vi "HEWH RLT Selected MW100 TCs.vi"(0 "Core HEWH Data Station A":T1={"Scan Rate Adjust"=0.0, "Draw Count"=0, "Test Patten Setup"={"Total Gallons Schedule"=[], "PRAT/RLT Sequence"=[{"Sequence #"=1.0, "Cycles"=35, "Mode Setting"="", "Flow Rate (GPM)"=0.0, "Temperature (F)"=0.0, "Reset Timer"=FALSE, "Use Temp Decline Method"=FALSE, "Terminate Condition"=enum."C1-Terminate Draw @ Gallon Mark", "Condition Value #1"=0.0, "UE"=FALSE, "LE"=FALSE, "Comp"=FALSE, "Fan"=FALSE, "Test End Time (Sec)"=0.0, "Purge Until Cutout"=FALSE, "Start Conditions"=enum."Heat Source Cutout", "Condition Value #2"=0.0, "Remove Power"=FALSE, "Time"=0.0, "Check Special Cond."=enum."SC2-Check Heat Source (On-C2/Off-C1)", "Condition#"=enum."C1", "Draw Flags"=enum."N/A", "Data Processing Delay (FHD 15sec, UEF 5 Sec)"=0.0, "Test Complete"=FALSE, "User Setpoint"=0.0, "Tank Setpoint"=0.0}, {"Sequence #"=2.0, "Cycles"=15, "Mode Setting"="", "Flow Rate (GPM)"=0.0, "Temperature (F)"=0.0, "Reset Timer"=FALSE, "Use Temp Decline Method"=FALSE, "Terminate Condition"=enum."C1-Terminate Draw @ Gallon Mark", "Condition Value #1"=0.0, "UE"=FALSE, "LE"=FALSE, "Comp"=FALSE, "Fan"=FALSE, "Test End Time (Sec)"=0.0, "Purge Until Cutout"=FALSE, "Start Conditions"=enum."Heat Source Cutout", "Condition Value #2"=0.0, "Remove Power"=FALSE, "Time"=0.0, "Check Special Cond."=enum."SC2-Check Heat Source (On-C2/Off-C1)", "Condition#"=enum."C1", "Draw Flags"=enum."N/A", "Data Processing Delay (FHD 15sec, UEF 5 Sec)"=0.0, "Test Complete"=FALSE, "User Setpoint"=0.0, "Tank Setpoint"=0.0}, {"Sequence #"=3.0, "Cycles"=35, "Mode Setting"="", "Flow Rate (GPM)"=0.0, "Temperature (F)"=0.0, "Reset Timer"=FALSE, "Use Temp Decline Method"=FALSE, "Terminate Condition"=enum."C1-Terminate Draw @ Gallon Mark", "Condition Value #1"=0.0, "UE"=FALSE, "LE"=FALSE, "Comp"=FALSE, "Fan"=FALSE, "Test End Time (Sec)"=0.0, "Purge Until Cutout"=FALSE, "Start Conditions"=enum."Heat Source Cutout", "Condition Value #2"=0.0, "Remove Power"=FALSE, "Time"=0.0, "Check Special Cond."=enum."SC2-Check Heat Source (On-C2/Off-C1)", "Condition#"=enum."C1", "Draw Flags"=enum."N/A", "Data Processing Delay (FHD 15sec, UEF 5 Sec)"=0.0, "Test Complete"=FALSE, "User Setpoint"=0.0, "Tank Setpoint"=0.0}, {"Sequence #"=4.0, "Cycles"=15, "Mode Setting"="", "Flow Rate (GPM)"=0.0, "Temperature (F)"=0.0, "Reset Timer"=FALSE, "Use Temp Decline Method"=FALSE, "Terminate Condition"=enum."C1-Terminate Draw @ Gallon Mark", "Condition Value #1"=0.0, "UE"=FALSE, "LE"=FALSE, "Comp"=FALSE, "Fan"=FALSE, "Test End Time (Sec)"=0.0, "Purge Until Cutout"=FALSE, "Start Conditions"=enum."Heat Source Cutout", "Condition Value #2"=0.0, "Remove Power"=FALSE, "Time"=0.0, "Check Special Cond."=enum."SC2-Check Heat Source (On-C2/Off-C1)", "Condition#"=enum."C1", "Draw Flags"=enum."N/A", "Data Processing Delay (FHD 15sec, UEF 5 Sec)"=0.0, "Test Complete"=FALSE, "User Setpoint"=0.0, "Tank Setpoint"=0.0}, {"Sequence #"=5.0, "Cycles"=35, "Mode Setting"="", "Flow Rate (GPM)"=0.0, "Temperature (F)"=0.0, "Reset Timer"=FALSE, "Use Temp Decline Method"=FALSE, "Terminate Condition"=enum."C1-Terminate Draw @ Gallon Mark", "Condition Value #1"=0.0, "UE"=FALSE, "LE"=FALSE, "Comp"=FALSE, "Fan"=FALSE, "Test End Time (Sec)"=0.0, "Purge Until Cutout"=FALSE, "Start Conditions"=enum."Heat Source Cutout", "Condition Value #2"=0.0, "Remove Power"=FALSE, "Time"=0.0, "Check Special Cond."=enum."SC2-Check Heat Source (On-C2/Off-C1)", "Condition#"=enum."C1", "Draw Flags"=enum."N/A", "Data Processing Delay (FHD 15sec, UEF 5 Sec)"=0.0, "Test Complete"=FALSE, "User Setpoint"=0.0, "Tank Setpoint"=0.0}, {"Sequence #"=6.0, "Cycles"=15, "Mode Setting"="", "Flow Rate (GPM)"=0.0, "Temperature (F)"=0.0, "Reset Timer"=FALSE, "Use Temp Decline Method"=FALSE, "Terminate Condition"=enum."C1-Terminate Draw @ Gallon Mark", "Condition Value #1"=0.0, "UE"=FALSE, "LE"=FALSE, "Comp"=FALSE, "Fan"=FALSE, "Test End Time (Sec)"=0.0, "Purge Until Cutout"=FALSE, "Start Conditions"=enum."Heat Source Cutout", "Condition Value #2"=0.0, "Remove Power"=FALSE, "Time"=0.0, "Check Special Cond."=enum."SC2-Check Heat Source (On-C2/Off-C1)", "Condition#"=enum."C1", "Draw Flags"=enum."N/A", "Data Processing Delay (FHD 15sec, UEF 5 Sec)"=0.0, "Test Complete"=FALSE, "User Setpoint"=0.0, "Tank Setpoint"=0.0}, {"Sequence #"=7.0, "Cycles"=35, "Mode Setting"="", "Flow Rate (GPM)"=0.0, "Temperature (F)"=0.0, "Reset Timer"=FALSE, "Use Temp Decline Method"=FALSE, "Terminate Condition"=enum."C1-Terminate Draw @ Gallon Mark", "Condition Value #1"=0.0, "UE"=FALSE, "LE"=FALSE, "Comp"=FALSE, "Fan"=FALSE, "Test End Time (Sec)"=0.0, "Purge Until Cutout"=FALSE, "Start Conditions"=enum."Heat Source Cutout", "Condition Value #2"=0.0, "Remove Power"=FALSE, "Time"=0.0, "Check Special Cond."=enum."SC2-Check Heat Source (On-C2/Off-C1)", "Condition#"=enum."C1", "Draw Flags"=enum."N/A", "Data Processing Delay (FHD 15sec, UEF 5 Sec)"=0.0, "Test Complete"=FALSE, "User Setpoint"=0.0, "Tank Setpoint"=0.0}, {"Sequence #"=8.0, "Cycles"=15, "Mode Setting"="", "Flow Rate (GPM)"=0.0, "Temperature (F)"=0.0, "Reset Timer"=FALSE, "Use Temp Decline Method"=FALSE, "Terminate Condition"=enum."C1-Terminate Draw @ Gallon Mark", "Condition Value #1"=0.0, "UE"=FALSE, "LE"=FALSE, "Comp"=FALSE, "Fan"=FALSE, "Test End Time (Sec)"=0.0, "Purge Until Cutout"=FALSE, "Start Conditions"=enum."Heat Source Cutout", "Condition Value #2"=0.0, "Remove Power"=FALSE, "Time"=0.0, "Check Special Cond."=enum."SC2-Check Heat Source (On-C2/Off-C1)", "Condition#"=enum."C1", "Draw Flags"=enum."N/A", "Data Processing Delay (FHD 15sec, UEF 5 Sec)"=0.0, "Test Complete"=FALSE, "User Setpoint"=0.0, "Tank Setpoint"=0.0}], "Current Sequence Index"=0}, "HEWH Specific DAQ"={"HEWH Data"={"HEWH Standard"={"Voltage (Volts)"=0.0, "Current (Amps)"=0.0, "Power (Watts)"=0.0, "WattHours (Wh)"=0.0, "TC Tree (AVG)"=0.0, "Flow Rate (GPM)"=0.0, "Gallons (Gal)"=0.0, "RTD Out (Deg F)"=0.0, "RTD In (Deg F)"=0.0, "RTD Amb (Deg F)"=0.0, "TC Down"=0.0, "UE Event Lead"=0, "LE Event Lead"=0, "TC 8"=0.0, "TC 9"=0.0, "TC 10"=0.0, "TC Tree Array (1-6)"=[], "TC 7"=0.0, "PSI 1"=0.0, "PSI 2"=0.0, "PSI 3"=0.0, "PSI 4"=0.0}, "PRAT"={"Power (Watts) A"=4192.0, "Power (Watts) B"=4192.0, "Power (Watts) C"=4192.0, "Power (Watts) D"=4192.0, "TC1"=0.0, "TC2"=0.0, "TC3"=0.0, "TC4"=0.0, "WattHours (Wh) A"=4192.0, "WattHours (Wh) B"=4192.0, "WattHours (Wh) C"=4192.0, "WattHours (Wh) D"=4192.0, "Ambient"=0.0, "Extra Temp"=0.0}, "Additional Power Data"={"Vthd"=236.2, "Frequency (Hz)"=236.2, "Apparent Power (VA)"=236.2, "Power Factor"=236.2, "Current Crest Factor"=236.2, "Voltage Crest Factor"=236.2, "Integration Time (sec)"=236.2}}, "Flow Valve % Open"=0.0, "Power State"={"UE"=FALSE, "LE"=FALSE, "COMP"=FALSE, "FANS"=FALSE}, "Power Analyzer"=enum."APLUS", "Flow Valve uA Output"=0, "Gallons Start (Gal)"=0.0, "PI Output"=0.0}, "Test Output Data"={"PreDraw Data Table"=[], "Data Table"=[], "MW100 TC Headers"=[]}, "Calc and Calibration"={"Mean SD Var Max Min Array"=[], "Draw Statistics (DBL)"=[], "Calibration Coefficients DBL"=[], "Start Gallons"=0.0, "Starting Temp Decline"=0.0, "K-Factor (Temperature)"=0.0, "All Draw Stats"=[], "RTD Terminate Value"=0.0, "K-Factor (Flow)"=0.0, "Intellifaucet Type"="", "Thermal Stabil Array"=[], "Gas Thermal Stabil Complete"=FALSE, "Therm Reset Cmpt 1"=FALSE, "Therm Reset Cmpt 2"=FALSE, "Last Flow Rate (Therm)"=0.0, "State"=enum."State 1", "Gas Thermal Time"=0.0, "Target Rate (Thermal)"=0.0, "Thermal - Final"=[], "State5 Gal Water"=0.0, "State 5 Gal Gas"=0.0, "Intellif Open < 1"=0.0, "Intellif Open < 1.7"=0.0, "Intellif Open < 2.2"=0.0, "Intellif Open > 2.2"=0.0, "End of Draw\nComparison"=[], "Temperature Decline Method"={"Previous Cycle Count"=0, "Previous Max Temp In"=0.0, "Previous Trigger In"=0, "Start Timer"=0.0, "first_iteration"=0.0}}, "Current Draw Time"=0.0, "LV Program"=enum."HEWH", "Station ID"=enum."A", "Current Cond"=enum."N/A", "Test Complete"=FALSE, "ANSI Rate"={"Array 1"=[], "Array 3"=[], "Array 2"=[], "Start ANSI"=FALSE, "ANSI Start Time"=0.0, "Restart ANSI"=FALSE, "15 Min ANSI Avg (BTU/hr)"=0.0, "20 Min ANSI Avg (BTU/hr)"=0.0, "25 Min ANSI Avg (BTU/hr)"=0.0, "Absolute Pressure"=0.0, "Gas Temperature"=0.0, "Volumetric Flow Rate"=0.0, "Mass Flow Rate"=0.0, "Array 4"=[], "Array 5"=[], "Gas Rate"=0.0, "15 Min Pres Avg (PSIA)"=0.0, "20 Min Pres Avg (PSIA)"=0.0, "25 Min Pres Avg (PSIA)"=0.0, "15 Min Temp Avg (°F) "=0.0, "20 Min Temp Avg (°F)"=0.0, "25 Min Temp Avg (°F)"=0.0, "15 Min Uncorrected Avg (CFH)"=0.0, "20 Min Uncorrected Avg (CFH)"=0.0, "25 Min Uncorrected Avg (CFH)"=0.0, "15 Min Corrected Avg (SCFH)"=0.0, "20 Min Corrected Avg (SCFH)"=0.0, "25 Min Corrected Avg (SCFH)"=0.0, "15 Min Complete"=FALSE, "20 Min Complete"=FALSE, "25 Min Complete"=FALSE, "Heating Value (BTU/ft³)"=0.0, "CO CO2 15 Min"=[], "CO CO2 20 Min"=[], "CO CO2 25 Min"=[], "CO CO2 Real Time"=[]}, "Module 4 Relay Status"={"INTELLIFAUCET TEMP(T)/FLOW(F) (CH 041)"=FALSE, "INTELLIFAUCET READY (CH 042)"=FALSE, "INTELLIFAUCET START (CH 043)"=FALSE, "INTELLIFAUCET STOP (CH 044)"=FALSE, "MAIN POWER RELAY (CH 047)"=FALSE, "NOT USED (CH 045)"=FALSE, "NOT USED (CH 046)"=FALSE, "PURGE VALVE RELAY (CH 048)"=FALSE, "OUTLET VALVE RELAY (CH 049)"=FALSE, "INLET VALVE RELAY (CH 050)"=FALSE, "Intellifaucet (% Open)"=0.0, "Proportioning Valve (%Open)"=0.0, "Intellifaucet Temp Setpoint (F)"=0.0}} {"Test Patten Setup"."PRAT/RLT Sequence"."Time" format="%<%H:%M:%S>t"; "Test Patten Setup"."Total Gallons Schedule" format="%.2f"}, 1 "Current Drawing Station":string="A", 2 "Show Flow Data":bool, 9 "MW100 Full Data":string[][](array[string])=[["Voltage (V)", "0.000"], ["RMS Current (Amps)", "0.000"], ["Power (Watts)", "0.000"], ["Watt Hours (Wh)", "0.000"], ["Voltage Total Harmonic Distortion", "0.000"], ["Frequency (Hz)", "0.000"], ["Apparent Power (VA)", "0.000"], ["Power Factor", "0.000"], ["Current Crest Factor", "0.000"], ["Voltage Crest Factor", "0.000"], ["Integration Time (sec)", "0.000"], ["Intellifaucet Valve % Open", "0.000"], ["Draw Count", "1"], ["T1", "10.2"], ["T2", "20"], ["T3", "0.000"], ["T4", "0.000"], ["T5", "0.000"], ["T6", "0.000"], ["T7", "0.000"], ["T8", "0.000"], ["T9", "0.000"], ["T10", "0.000"], ["TC Tree Average", "0.000"], ["TC Down", "0.000"], ["RTD IN", "0.000"], ["RTD Out", "0.000"], ["RTD Ambient", "0.000"], ["Totalized Flow (Linear Link) - Calculated (Gallons)", "0.000"], ["Flow Rate (Linear Link) - Calculated (GPM)", "0.000"], ["Pressure - HI1", "0.000"], ["Pressure - HI2", "0.000"], ["Pressure - LOW", "0.000"], ["Pressure - PIN", "0.000"]], 11 "Error In":errorcluster, 12 "Station A Channels, MW100":string[][](array[string])=[["T1 - IN", "11"], ["T1 - OUT", "13"]], 13 "Station ID":string="A", 14 "Collect Power Data":bool) -> (3 "Data (Label,Data)":string[][](array[string])=[["Voltage (V)", "0.000"], ["RMS Current (Amps)", "0.000"], ["Power (Watts)", "0.000"], ["Watt Hours (Wh)", "0.000"], ["Voltage Total Harmonic Distortion", "0.000"], ["Frequency (Hz)", "0.000"], ["Apparent Power (VA)", "0.000"], ["Power Factor", "0.000"], ["Current Crest Factor", "0.000"], ["Voltage Crest Factor", "0.000"], ["Integration Time (sec)", "0.000"], ["Intellifaucet Valve % Open", "0.000"], ["TC Tree Average", "0.000"], ["TC Down", "0.000"], ["RTD IN", "0.000"], ["RTD Out", "0.000"], ["RTD Ambient", "0.000"], ["Totalized Flow (Linear Link) - Calculated (Gallons)", "0.000"], ["Flow Rate (Linear Link) - Calculated (GPM)", "0.000"], ["Pressure - HI1", "0.000"], ["Pressure - HI2", "0.000"], ["Pressure - LOW", "0.000"], ["Pressure - PIN", "0.000"]], 4 "Core HEWH Data Station Output":T1={"Scan Rate Adjust"=0.0, "Draw Count"=0, "Test Patten Setup"={"Total Gallons Schedule"=[], "PRAT/RLT Sequence"=[{"Sequence #"=1.0, "Cycles"=35, "Mode Setting"="", "Flow Rate (GPM)"=0.0, "Temperature (F)"=0.0, "Reset Timer"=FALSE, "Use Temp Decline Method"=FALSE, "Terminate Condition"=enum."C1-Terminate Draw @ Gallon Mark", "Condition Value #1"=0.0, "UE"=FALSE, "LE"=FALSE, "Comp"=FALSE, "Fan"=FALSE, "Test End Time (Sec)"=0.0, "Purge Until Cutout"=FALSE, "Start Conditions"=enum."Heat Source Cutout", "Condition Value #2"=0.0, "Remove Power"=FALSE, "Time"=0.0, "Check Special Cond."=enum."SC2-Check Heat Source (On-C2/Off-C1)", "Condition#"=enum."C1", "Draw Flags"=enum."N/A", "Data Processing Delay (FHD 15sec, UEF 5 Sec)"=0.0, "Test Complete"=FALSE, "User Setpoint"=0.0, "Tank Setpoint"=0.0}, {"Sequence #"=2.0, "Cycles"=15, "Mode Setting"="", "Flow Rate (GPM)"=0.0, "Temperature (F)"=0.0, "Reset Timer"=FALSE, "Use Temp Decline Method"=FALSE, "Terminate Condition"=enum."C1-Terminate Draw @ Gallon Mark", "Condition Value #1"=0.0, "UE"=FALSE, "LE"=FALSE, "Comp"=FALSE, "Fan"=FALSE, "Test End Time (Sec)"=0.0, "Purge Until Cutout"=FALSE, "Start Conditions"=enum."Heat Source Cutout", "Condition Value #2"=0.0, "Remove Power"=FALSE, "Time"=0.0, "Check Special Cond."=enum."SC2-Check Heat Source (On-C2/Off-C1)", "Condition#"=enum."C1", "Draw Flags"=enum."N/A", "Data Processing Delay (FHD 15sec, UEF 5 Sec)"=0.0, "Test Complete"=FALSE, "User Setpoint"=0.0, "Tank Setpoint"=0.0}, {"Sequence #"=3.0, "Cycles"=35, "Mode Setting"="", "Flow Rate (GPM)"=0.0, "Temperature (F)"=0.0, "Reset Timer"=FALSE, "Use Temp Decline Method"=FALSE, "Terminate Condition"=enum."C1-Terminate Draw @ Gallon Mark", "Condition Value #1"=0.0, "UE"=FALSE, "LE"=FALSE, "Comp"=FALSE, "Fan"=FALSE, "Test End Time (Sec)"=0.0, "Purge Until Cutout"=FALSE, "Start Conditions"=enum."Heat Source Cutout", "Condition Value #2"=0.0, "Remove Power"=FALSE, "Time"=0.0, "Check Special Cond."=enum."SC2-Check Heat Source (On-C2/Off-C1)", "Condition#"=enum."C1", "Draw Flags"=enum."N/A", "Data Processing Delay (FHD 15sec, UEF 5 Sec)"=0.0, "Test Complete"=FALSE, "User Setpoint"=0.0, "Tank Setpoint"=0.0}, {"Sequence #"=4.0, "Cycles"=15, "Mode Setting"="", "Flow Rate (GPM)"=0.0, "Temperature (F)"=0.0, "Reset Timer"=FALSE, "Use Temp Decline Method"=FALSE, "Terminate Condition"=enum."C1-Terminate Draw @ Gallon Mark", "Condition Value #1"=0.0, "UE"=FALSE, "LE"=FALSE, "Comp"=FALSE, "Fan"=FALSE, "Test End Time (Sec)"=0.0, "Purge Until Cutout"=FALSE, "Start Conditions"=enum."Heat Source Cutout", "Condition Value #2"=0.0, "Remove Power"=FALSE, "Time"=0.0, "Check Special Cond."=enum."SC2-Check Heat Source (On-C2/Off-C1)", "Condition#"=enum."C1", "Draw Flags"=enum."N/A", "Data Processing Delay (FHD 15sec, UEF 5 Sec)"=0.0, "Test Complete"=FALSE, "User Setpoint"=0.0, "Tank Setpoint"=0.0}, {"Sequence #"=5.0, "Cycles"=35, "Mode Setting"="", "Flow Rate (GPM)"=0.0, "Temperature (F)"=0.0, "Reset Timer"=FALSE, "Use Temp Decline Method"=FALSE, "Terminate Condition"=enum."C1-Terminate Draw @ Gallon Mark", "Condition Value #1"=0.0, "UE"=FALSE, "LE"=FALSE, "Comp"=FALSE, "Fan"=FALSE, "Test End Time (Sec)"=0.0, "Purge Until Cutout"=FALSE, "Start Conditions"=enum."Heat Source Cutout", "Condition Value #2"=0.0, "Remove Power"=FALSE, "Time"=0.0, "Check Special Cond."=enum."SC2-Check Heat Source (On-C2/Off-C1)", "Condition#"=enum."C1", "Draw Flags"=enum."N/A", "Data Processing Delay (FHD 15sec, UEF 5 Sec)"=0.0, "Test Complete"=FALSE, "User Setpoint"=0.0, "Tank Setpoint"=0.0}, {"Sequence #"=6.0, "Cycles"=15, "Mode Setting"="", "Flow Rate (GPM)"=0.0, "Temperature (F)"=0.0, "Reset Timer"=FALSE, "Use Temp Decline Method"=FALSE, "Terminate Condition"=enum."C1-Terminate Draw @ Gallon Mark", "Condition Value #1"=0.0, "UE"=FALSE, "LE"=FALSE, "Comp"=FALSE, "Fan"=FALSE, "Test End Time (Sec)"=0.0, "Purge Until Cutout"=FALSE, "Start Conditions"=enum."Heat Source Cutout", "Condition Value #2"=0.0, "Remove Power"=FALSE, "Time"=0.0, "Check Special Cond."=enum."SC2-Check Heat Source (On-C2/Off-C1)", "Condition#"=enum."C1", "Draw Flags"=enum."N/A", "Data Processing Delay (FHD 15sec, UEF 5 Sec)"=0.0, "Test Complete"=FALSE, "User Setpoint"=0.0, "Tank Setpoint"=0.0}, {"Sequence #"=7.0, "Cycles"=35, "Mode Setting"="", "Flow Rate (GPM)"=0.0, "Temperature (F)"=0.0, "Reset Timer"=FALSE, "Use Temp Decline Method"=FALSE, "Terminate Condition"=enum."C1-Terminate Draw @ Gallon Mark", "Condition Value #1"=0.0, "UE"=FALSE, "LE"=FALSE, "Comp"=FALSE, "Fan"=FALSE, "Test End Time (Sec)"=0.0, "Purge Until Cutout"=FALSE, "Start Conditions"=enum."Heat Source Cutout", "Condition Value #2"=0.0, "Remove Power"=FALSE, "Time"=0.0, "Check Special Cond."=enum."SC2-Check Heat Source (On-C2/Off-C1)", "Condition#"=enum."C1", "Draw Flags"=enum."N/A", "Data Processing Delay (FHD 15sec, UEF 5 Sec)"=0.0, "Test Complete"=FALSE, "User Setpoint"=0.0, "Tank Setpoint"=0.0}, {"Sequence #"=8.0, "Cycles"=15, "Mode Setting"="", "Flow Rate (GPM)"=0.0, "Temperature (F)"=0.0, "Reset Timer"=FALSE, "Use Temp Decline Method"=FALSE, "Terminate Condition"=enum."C1-Terminate Draw @ Gallon Mark", "Condition Value #1"=0.0, "UE"=FALSE, "LE"=FALSE, "Comp"=FALSE, "Fan"=FALSE, "Test End Time (Sec)"=0.0, "Purge Until Cutout"=FALSE, "Start Conditions"=enum."Heat Source Cutout", "Condition Value #2"=0.0, "Remove Power"=FALSE, "Time"=0.0, "Check Special Cond."=enum."SC2-Check Heat Source (On-C2/Off-C1)", "Condition#"=enum."C1", "Draw Flags"=enum."N/A", "Data Processing Delay (FHD 15sec, UEF 5 Sec)"=0.0, "Test Complete"=FALSE, "User Setpoint"=0.0, "Tank Setpoint"=0.0}], "Current Sequence Index"=0}, "HEWH Specific DAQ"={"HEWH Data"={"HEWH Standard"={"Voltage (Volts)"=0.0, "Current (Amps)"=0.0, "Power (Watts)"=0.0, "WattHours (Wh)"=0.0, "TC Tree (AVG)"=0.0, "Flow Rate (GPM)"=0.0, "Gallons (Gal)"=0.0, "RTD Out (Deg F)"=0.0, "RTD In (Deg F)"=0.0, "RTD Amb (Deg F)"=0.0, "TC Down"=0.0, "UE Event Lead"=0, "LE Event Lead"=0, "TC 8"=0.0, "TC 9"=0.0, "TC 10"=0.0, "TC Tree Array (1-6)"=[], "TC 7"=0.0, "PSI 1"=0.0, "PSI 2"=0.0, "PSI 3"=0.0, "PSI 4"=0.0}, "PRAT"={"Power (Watts) A"=4192.0, "Power (Watts) B"=4192.0, "Power (Watts) C"=4192.0, "Power (Watts) D"=4192.0, "TC1"=0.0, "TC2"=0.0, "TC3"=0.0, "TC4"=0.0, "WattHours (Wh) A"=4192.0, "WattHours (Wh) B"=4192.0, "WattHours (Wh) C"=4192.0, "WattHours (Wh) D"=4192.0, "Ambient"=0.0, "Extra Temp"=0.0}, "Additional Power Data"={"Vthd"=236.2, "Frequency (Hz)"=236.2, "Apparent Power (VA)"=236.2, "Power Factor"=236.2, "Current Crest Factor"=236.2, "Voltage Crest Factor"=236.2, "Integration Time (sec)"=236.2}}, "Flow Valve % Open"=0.0, "Power State"={"UE"=FALSE, "LE"=FALSE, "COMP"=FALSE, "FANS"=FALSE}, "Power Analyzer"=enum."APLUS", "Flow Valve uA Output"=0, "Gallons Start (Gal)"=0.0, "PI Output"=0.0}, "Test Output Data"={"PreDraw Data Table"=[], "Data Table"=[], "MW100 TC Headers"=[]}, "Calc and Calibration"={"Mean SD Var Max Min Array"=[], "Draw Statistics (DBL)"=[], "Calibration Coefficients DBL"=[], "Start Gallons"=0.0, "Starting Temp Decline"=0.0, "K-Factor (Temperature)"=0.0, "All Draw Stats"=[], "RTD Terminate Value"=0.0, "K-Factor (Flow)"=0.0, "Intellifaucet Type"="", "Thermal Stabil Array"=[], "Gas Thermal Stabil Complete"=FALSE, "Therm Reset Cmpt 1"=FALSE, "Therm Reset Cmpt 2"=FALSE, "Last Flow Rate (Therm)"=0.0, "State"=enum."State 1", "Gas Thermal Time"=0.0, "Target Rate (Thermal)"=0.0, "Thermal - Final"=[], "State5 Gal Water"=0.0, "State 5 Gal Gas"=0.0, "Intellif Open < 1"=0.0, "Intellif Open < 1.7"=0.0, "Intellif Open < 2.2"=0.0, "Intellif Open > 2.2"=0.0, "End of Draw\nComparison"=[], "Temperature Decline Method"={"Previous Cycle Count"=0, "Previous Max Temp In"=0.0, "Previous Trigger In"=0, "Start Timer"=0.0, "first_iteration"=0.0}}, "Current Draw Time"=0.0, "LV Program"=enum."HEWH", "Station ID"=enum."A", "Current Cond"=enum."N/A", "Test Complete"=FALSE, "ANSI Rate"={"Array 1"=[], "Array 3"=[], "Array 2"=[], "Start ANSI"=FALSE, "ANSI Start Time"=0.0, "Restart ANSI"=FALSE, "15 Min ANSI Avg (BTU/hr)"=0.0, "20 Min ANSI Avg (BTU/hr)"=0.0, "25 Min ANSI Avg (BTU/hr)"=0.0, "Absolute Pressure"=0.0, "Gas Temperature"=0.0, "Volumetric Flow Rate"=0.0, "Mass Flow Rate"=0.0, "Array 4"=[], "Array 5"=[], "Gas Rate"=0.0, "15 Min Pres Avg (PSIA)"=0.0, "20 Min Pres Avg (PSIA)"=0.0, "25 Min Pres Avg (PSIA)"=0.0, "15 Min Temp Avg (°F) "=0.0, "20 Min Temp Avg (°F)"=0.0, "25 Min Temp Avg (°F)"=0.0, "15 Min Uncorrected Avg (CFH)"=0.0, "20 Min Uncorrected Avg (CFH)"=0.0, "25 Min Uncorrected Avg (CFH)"=0.0, "15 Min Corrected Avg (SCFH)"=0.0, "20 Min Corrected Avg (SCFH)"=0.0, "25 Min Corrected Avg (SCFH)"=0.0, "15 Min Complete"=FALSE, "20 Min Complete"=FALSE, "25 Min Complete"=FALSE, "Heating Value (BTU/ft³)"=0.0, "CO CO2 15 Min"=[], "CO CO2 20 Min"=[], "CO CO2 25 Min"=[], "CO CO2 Real Time"=[]}, "Module 4 Relay Status"={"INTELLIFAUCET TEMP(T)/FLOW(F) (CH 041)"=FALSE, "INTELLIFAUCET READY (CH 042)"=FALSE, "INTELLIFAUCET START (CH 043)"=FALSE, "INTELLIFAUCET STOP (CH 044)"=FALSE, "MAIN POWER RELAY (CH 047)"=FALSE, "NOT USED (CH 045)"=FALSE, "NOT USED (CH 046)"=FALSE, "PURGE VALVE RELAY (CH 048)"=FALSE, "OUTLET VALVE RELAY (CH 049)"=FALSE, "INLET VALVE RELAY (CH 050)"=FALSE, "Intellifaucet (% Open)"=0.0, "Proportioning Valve (%Open)"=0.0, "Intellifaucet Temp Setpoint (F)"=0.0}} {"Test Patten Setup"."PRAT/RLT Sequence"."Time" format="%<%H:%M:%S>t"; "Test Patten Setup"."Total Gallons Schedule" format="%.2f"}, 8 "RMS Current (Amps)":dbl, 10 "TC Data":string[][](array[string]), 15 "Error Out":errorcluster)   [LabVIEW 2023]
uses:
  Type Definitions/HEWH Output Information.ctl
  Type Definitions/HEWH Draw Pattern Setup.ctl
  Type Definitions/PRAT Test.ctl
  Utility/Save File/File Setup (Public)/Type Definition/Save File HEWH Heating Control Mode.ctl
  Draw Water Specific/Type Definitions/Terminate Draw Conditions.ctl
  Type Definitions/HEWH Start Conditions.ctl
  Draw Water Specific/Type Definitions/Check Special Condtions.ctl
  Draw Water Specific/Type Definitions/HEWH Special Condition Check.ctl
  Type Definitions/HEWH Draw Flag ENUM.ctl
  Type Definitions/HEWH Specific DAQ.ctl
  Type Definitions/HEWH Power Data.ctl
  Type Definitions/HEWH Power Elements.ctl
  Utility/Type Definitions/UTILITY Power Analyzer.ctl
  Type Definitions/HEWH Calc and Calibration.ctl
  Utility/Save File/File Setup (Public)/Type Definition/Save File DOE LabView Program.ctl
  Custom Instrument Control/MW100/Type Definitions/Station ID Selector.ctl
  Range/Type Definitions/RANGE ANSI Rate.ctl
  Custom Instrument Control/MW100/Type Definitions/HEWH Module 4 Relay Status.ctl
  Type Definitions/PRAT Channel Settings.ctl
  Custom Instrument Control/MW100/Type Definitions/HEWH MW100 Channel Numbers.ctl
  Utility/Save File/File Setup.lvlib
panel:
  out "All Other Data (NO TC's)":string[][](array[string])
  in  "PRAT Example Data":string[][](array[string])=[["Power (Watts) - Station A", "1"], ["Power (Watts) - Station B", "2"], ["Power (Watts) - Station C", "3"], ["Power (Watts) - Station D", "4"], ["WattHours (Wh) - Station A", "1"], ["WattHours (Wh) - Station B", "2"], ["WattHours (Wh) - Station C", "3"], ["WattHours (Wh) - Station D", "4"], ["T1", "1"], ["T2", "2"], ["T3", "3"], ["T4", "4"], ["Ambient Temperature", "100"], ["Extra Temperature", "200"], ["Draw Count", "1"], ["Program Status", "Testing B..."]]
  # "Draw Pattern Setup (24 Hour)"
  # "Draw Pattern Setup (24 Hour)"
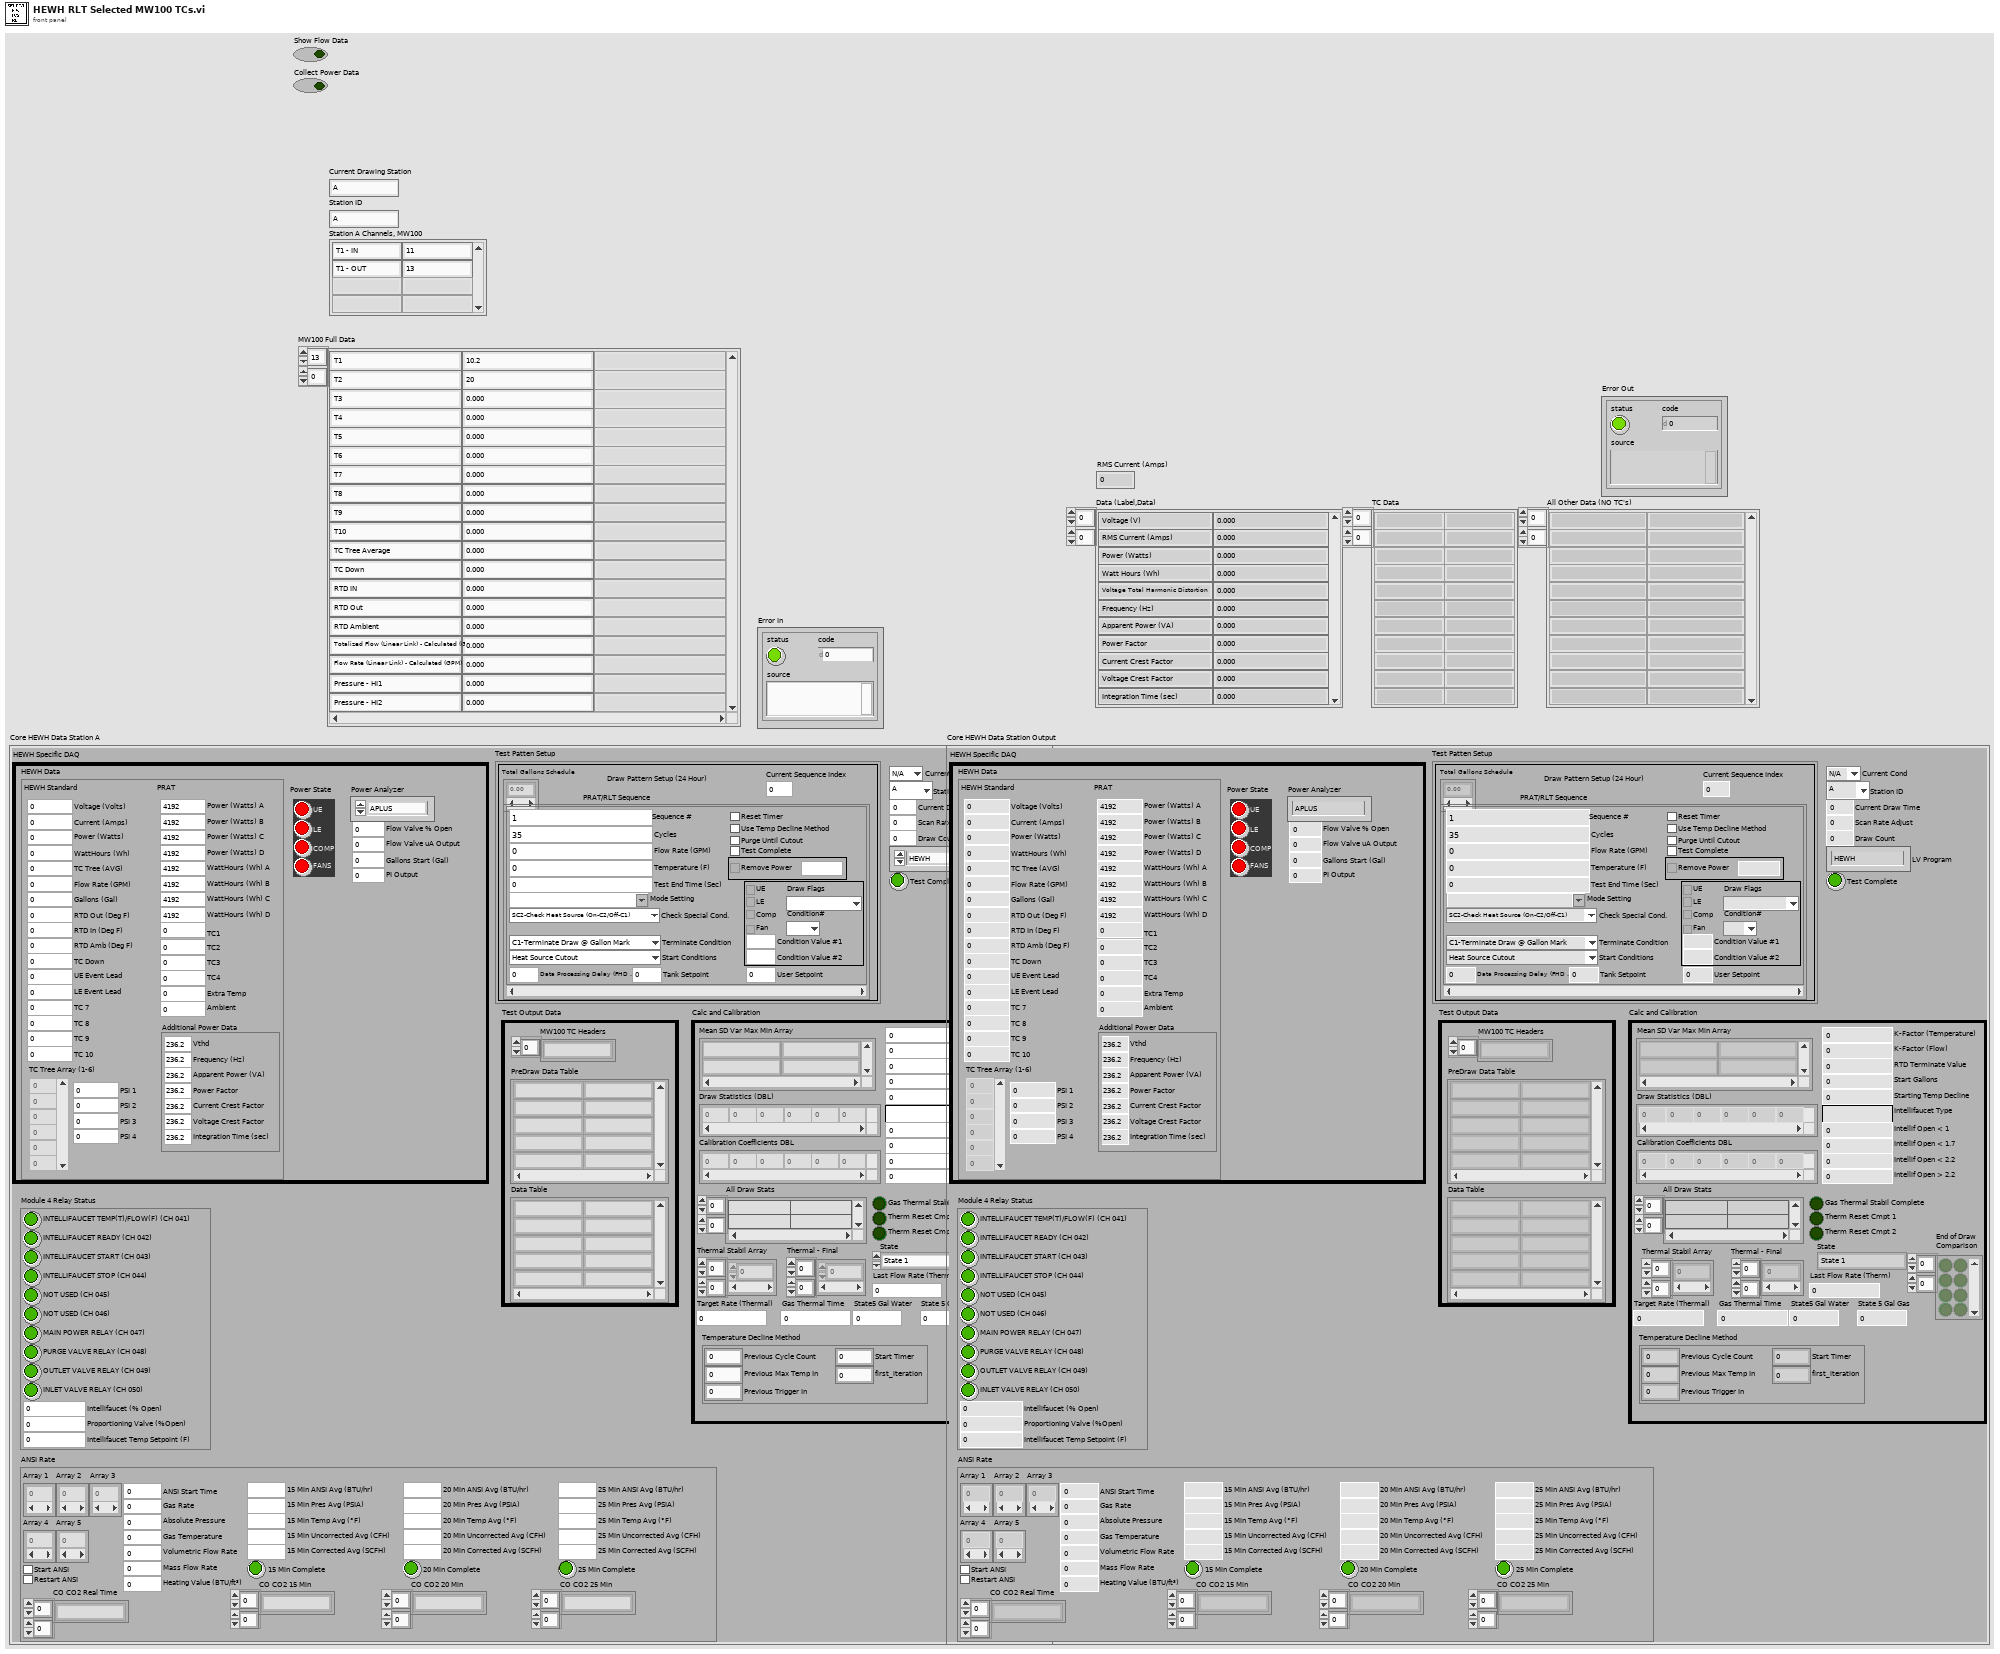
[diagram p1: front panel]
types:
  T1 = typedef "HEWH Output Information.ctl" = cluster{"Scan Rate Adjust":dbl, "Draw Count":i32, "Test Patten Setup":T2, "HEWH Specific DAQ":T10, "Test Output Data":cluster{"PreDraw Data Table":string[][], "Data Table":string[][], "MW100 TC Headers":string[]}, "Calc and Calibration":T14, "Current Draw Time":dbl, "LV Program":T15, "Station ID":T16, "Current Cond":T8, "Test Complete":bool, "ANSI Rate":T17, "Module 4 Relay Status":T18}
  T2 = typedef "HEWH Draw Pattern Setup.ctl" = cluster{"Total Gallons Schedule":dbl[], "PRAT/RLT Sequence":T3[], "Current Sequence Index":i32}
  T3 = typedef "PRAT Test.ctl" = cluster{"Sequence #":dbl, "Cycles":i32, "Mode Setting":T4, "Flow Rate (GPM)":dbl, "Temperature (F)":dbl, "Reset Timer":bool, "Use Temp Decline Method":bool, "Terminate Condition":T5, "Condition Value #1":dbl, "UE":bool, "LE":bool, "Comp":bool, "Fan":bool, "Test End Time (Sec)":dbl, "Purge Until Cutout":bool, "Start Conditions":T6, "Condition Value #2":dbl, "Remove Power":bool, "Time":dbl, "Check Special Cond.":T7, "Condition#":T8, "Draw Flags":T9, "Data Processing Delay (FHD 15sec, UEF 5 Sec)":dbl, "Test Complete":bool, "User Setpoint":dbl, "Tank Setpoint":dbl}
  T4 = typedef "File Setup.lvlib/Save File HEWH Heating Control Mode.ctl" = string
  T5 = typedef "Terminate Draw Conditions.ctl" = enum16{"C1-Terminate Draw @ Gallon Mark", "C2-Special Last Draw (HU Test)", "C3-RTD Out <=", "C4-Mean Tank Temp <=", "C5-Decrease RTD Out (Deg F)", "C6-Time (Seconds)", "C7-Until Any Heat Source", "C8-Specific Heat Source", "C9-Do Nothing", "C10-Inlet Outlet RTD Temp Delta"}
  T6 = typedef "HEWH Start Conditions.ctl" = enum16{"Heat Source Cutout", "At Time (Seconds)", "Every X (Seconds)", "T2 >= X° Below Setpoint", "Seconds From Complete", "Wait for LE & Comp Cutout", "Wait for Comp Cutout", "Wait for LE Cutout", "Wait for UE Cutout", "Start Immediately"}
  T7 = typedef "Check Special Condtions.ctl" = enum16{"SC1-Do Nothing", "SC2-Check Heat Source (On-C2/Off-C1)", "SC3-Check Skip Condition", "SC4-Check Heat Source ON/Fail", "SC5-Keep Draw Valves Open", "SC6-Skip Purge"}
  T8 = typedef "HEWH Special Condition Check.ctl" = enum16{"N/A", "C1", "C2", "Reset/Fail", "Skip Draw Sequence"}
  T9 = typedef "HEWH Draw Flag ENUM.ctl" = enum16{"N/A", "None(0)", "Sml(1)", "Med(2)", "SmlMed(3)", "Lrg(4)", "SmlLrg(5)", "MedLrg(6)", "SmlMedLrg(7)"}
  T10 = typedef "HEWH Specific DAQ.ctl" = cluster{"HEWH Data":T11, "Flow Valve % Open":dbl, "Power State":T12, "Power Analyzer":T13, "Flow Valve uA Output":i32, "Gallons Start (Gal)":dbl, "PI Output":dbl}
  T11 = typedef "HEWH Power Data.ctl" = cluster{"HEWH Standard":cluster{"Voltage (Volts)":dbl, "Current (Amps)":dbl, "Power (Watts)":dbl, "WattHours (Wh)":dbl, "TC Tree (AVG)":dbl, "Flow Rate (GPM)":dbl, "Gallons (Gal)":dbl, "RTD Out (Deg F)":dbl, "RTD In (Deg F)":dbl, "RTD Amb (Deg F)":dbl, "TC Down":dbl, "UE Event Lead":i32, "LE Event Lead":i32, "TC 8":dbl, "TC 9":dbl, "TC 10":dbl, "TC Tree Array (1-6)":dbl[], "TC 7":dbl, "PSI 1":dbl, "PSI 2":dbl, "PSI 3":dbl, "PSI 4":dbl}, "PRAT":cluster{"Power (Watts) A":dbl, "Power (Watts) B":dbl, "Power (Watts) C":dbl, "Power (Watts) D":dbl, "TC1":dbl, "TC2":dbl, "TC3":dbl, "TC4":dbl, "WattHours (Wh) A":dbl, "WattHours (Wh) B":dbl, "WattHours (Wh) C":dbl, "WattHours (Wh) D":dbl, "Ambient":dbl, "Extra Temp":dbl}, "Additional Power Data":cluster{"Vthd":dbl, "Frequency (Hz)":dbl, "Apparent Power (VA)":dbl, "Power Factor":dbl, "Current Crest Factor":dbl, "Voltage Crest Factor":dbl, "Integration Time (sec)":dbl}}
  T12 = typedef "HEWH Power Elements.ctl" = cluster{"UE":bool, "LE":bool, "COMP":bool, "FANS":bool}
  T13 = typedef "UTILITY Power Analyzer.ctl" = enum16{"", "APLUS", "WT210", "WT500", "WT300", "OSI", "Debug", "WT230", "WT300_1", "WT300_2"}
  T14 = typedef "HEWH Calc and Calibration.ctl" = cluster{"Mean SD Var Max Min Array":string[][], "Draw Statistics (DBL)":dbl[][], "Calibration Coefficients DBL":dbl[][], "Start Gallons":dbl, "Starting Temp Decline":dbl, "K-Factor (Temperature)":dbl, "All Draw Stats":string[][], "RTD Terminate Value":dbl, "K-Factor (Flow)":dbl, "Intellifaucet Type":string, "Thermal Stabil Array":dbl[][], "Gas Thermal Stabil Complete":bool, "Therm Reset Cmpt 1":bool, "Therm Reset Cmpt 2":bool, "Last Flow Rate (Therm)":dbl, "State":enum16{"State 0", "State 1", "State 2", "State 3", "State 4", "State 5", "State 6"}, "Gas Thermal Time":dbl, "Target Rate (Thermal)":dbl, "Thermal - Final":dbl[][], "State5 Gal Water":dbl, "State 5 Gal Gas":dbl, "Intellif Open < 1":dbl, "Intellif Open < 1.7":dbl, "Intellif Open < 2.2":dbl, "Intellif Open > 2.2":dbl, "End of Draw\nComparison":bool[][], "Temperature Decline Method":cluster{"Previous Cycle Count":i32, "Previous Max Temp In":dbl, "Previous Trigger In":u8, "Start Timer":dbl, "first_iteration":dbl}}
  T15 = typedef "File Setup.lvlib/Save File DOE LabView Program.ctl" = enum16{"No Name Found", "DOE Stand", "Dishwasher Kitchen", "Portable Stand", "HEWH", "Dryer", "Dryer WILT", "HCC", "PRAT", "HEWH RLT", "Refrigeration", "Gas Water Heater"}
  T16 = typedef "Station ID Selector.ctl" = enum16{"", "A", "B", "C", "D", "Global"}
  T17 = typedef "RANGE ANSI Rate.ctl" = cluster{"Array 1":dbl[], "Array 3":dbl[], "Array 2":dbl[], "Start ANSI":bool, "ANSI Start Time":dbl, "Restart ANSI":bool, "15 Min ANSI Avg (BTU/hr)":dbl, "20 Min ANSI Avg (BTU/hr)":dbl, "25 Min ANSI Avg (BTU/hr)":dbl, "Absolute Pressure":dbl, "Gas Temperature":dbl, "Volumetric Flow Rate":dbl, "Mass Flow Rate":dbl, "Array 4":dbl[], "Array 5":dbl[], "Gas Rate":dbl, "15 Min Pres Avg (PSIA)":dbl, "20 Min Pres Avg (PSIA)":dbl, "25 Min Pres Avg (PSIA)":dbl, "15 Min Temp Avg (°F) ":dbl, "20 Min Temp Avg (°F)":dbl, "25 Min Temp Avg (°F)":dbl, "15 Min Uncorrected Avg (CFH)":dbl, "20 Min Uncorrected Avg (CFH)":dbl, "25 Min Uncorrected Avg (CFH)":dbl, "15 Min Corrected Avg (SCFH)":dbl, "20 Min Corrected Avg (SCFH)":dbl, "25 Min Corrected Avg (SCFH)":dbl, "15 Min Complete":bool, "20 Min Complete":bool, "25 Min Complete":bool, "Heating Value (BTU/ft³)":dbl, "CO CO2 15 Min":string[][], "CO CO2 20 Min":string[][], "CO CO2 25 Min":string[][], "CO CO2 Real Time":string[][]}
  T18 = typedef "HEWH Module 4 Relay Status.ctl" = cluster{"INTELLIFAUCET TEMP(T)/FLOW(F) (CH 041)":bool, "INTELLIFAUCET READY (CH 042)":bool, "INTELLIFAUCET START (CH 043)":bool, "INTELLIFAUCET STOP (CH 044)":bool, "MAIN POWER RELAY (CH 047)":bool, "NOT USED (CH 045)":bool, "NOT USED (CH 046)":bool, "PURGE VALVE RELAY (CH 048)":bool, "OUTLET VALVE RELAY (CH 049)":bool, "INLET VALVE RELAY (CH 050)":bool, "Intellifaucet (% Open)":dbl, "Proportioning Valve (%Open)":dbl, "Intellifaucet Temp Setpoint (F)":dbl}
  T19 = typedef "PRAT Channel Settings.ctl" = string
  T20 = typedef "HEWH MW100 Channel Numbers.ctl" = string
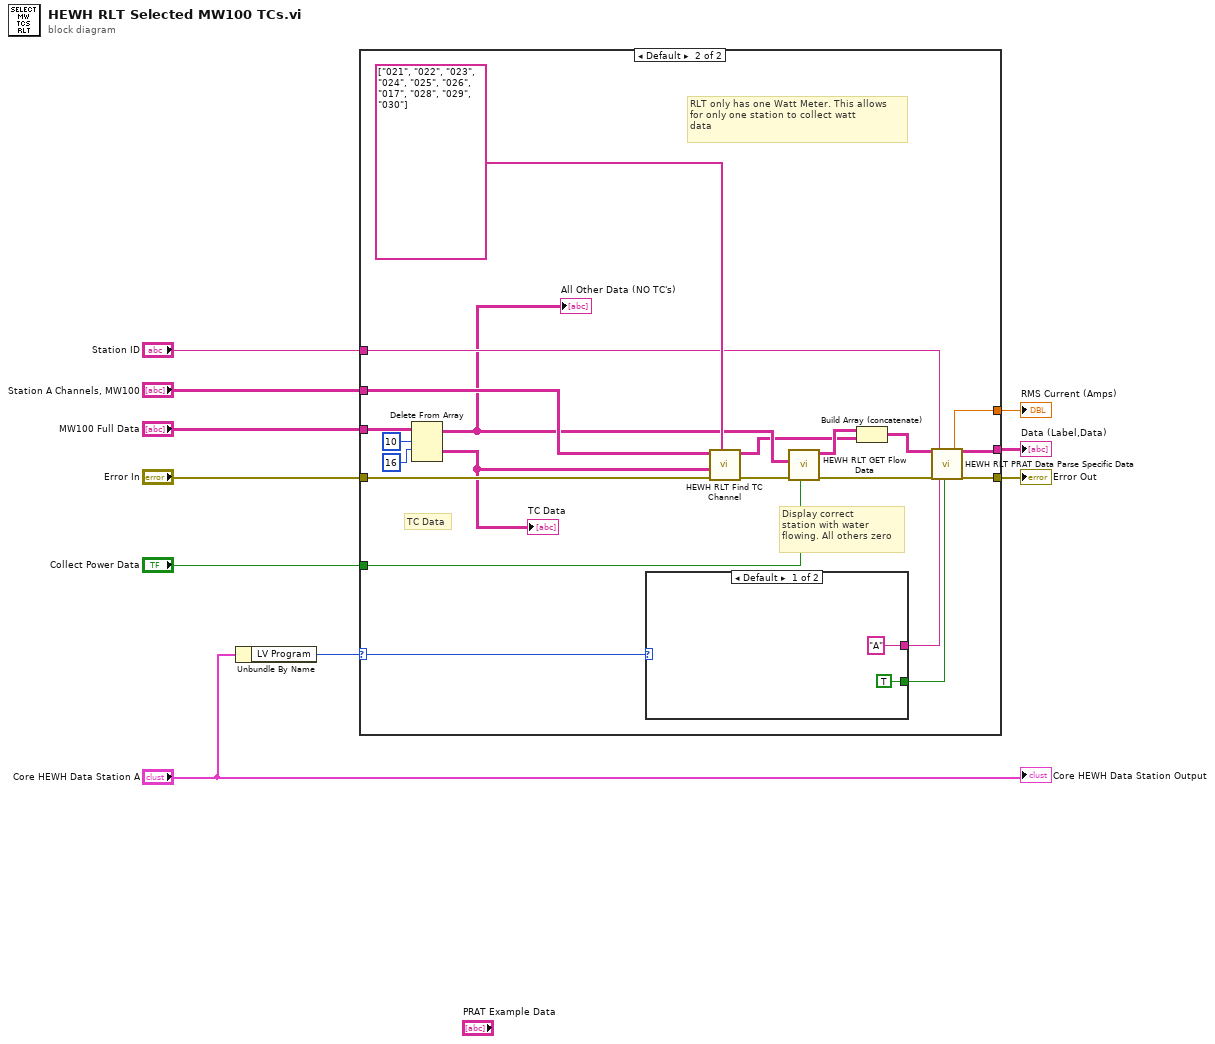
[diagram p0: block diagram]
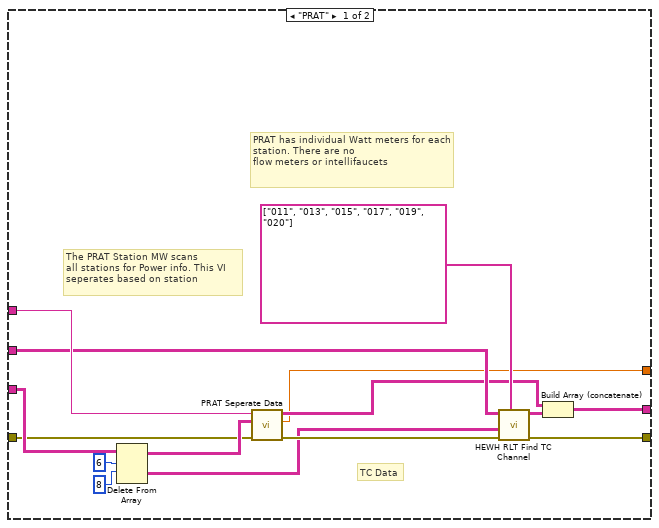
[diagram p2: hidden frame]
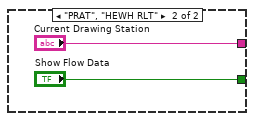
[diagram p3: hidden frame]
diagram:
  n1 = Unbundle By Name("Core HEWH Data Station A") -> ("LV Program"=w2:T15)
  n2 = case shown="Default" w2 {
    selector: w2 -> [_ w28]
    tunnel: "MW100 Full Data" -> [w23 w46]
    tunnel: "Station A Channels, MW100" -> [w15 w37]
    tunnel: [w12 w41] -> w10
    tunnel: "Error In" -> [w19 w42]
    tunnel: [w24 w40] -> w8
    tunnel: "Station ID" -> [w17 w39]
    tunnel: "Collect Power Data" -> [_ w30]
    tunnel: [w11 w27] -> w3
    frame "PRAT" {
      # "PRAT has individual Watt meters for each station. There are no\nflow meters or intellifaucets"
      # "The PRAT Station MW scans\nall stations for Power info. This VI\nseperates based on station"
      # "TC Data"
      n3 = Delete From Array(array=w23, length=6 ("index (row)"), index (row)=8) -> (deleted portion=w16:string[][], array with subset deleted=w21:string[][])  [unwired: 1 in]
      n4 = call "PRAT Seperate Data.vi"("Error In"=w19, "PRAT Power Data"=w21, "Prat Station"=w17) -> ("Error Out"=w18:errorcluster, "RMS Current (Amps)"=w11:dbl, "Station Power Data"=w14:string[][])  [unwired: 6 in]
      n5 = call "HEWH RLT Find TC Channel.vi"("Program Channel Locations In"=T19[] ["011", "013", "015", "017", "019", "020"], "Error In"=w18, "TC Data"=w16, "Station A Channels, MW100"=w15) -> ("Error Out"=w24:errorcluster, "TC Data"=w13:string[][])  [unwired: 6 in]
      n6 = Build Array (concatenate)(w14, w13) -> (w12:string[][])
    }
    frame Default {
      # "Display correct\nstation with water\nflowing. All others zero"
      # "RLT only has one Watt Meter. This allows\nfor only one station to collect watt \ndata"
      # "TC Data"
      n7 = Delete From Array(array=w46, length=10, index (row)=16 ("disabled index (row)")) -> (deleted portion=w38:string[][], array with subset deleted=w36:string[][])  [unwired: 1 in]
      "TC Data" <- w38
      "All Other Data (NO TC's)" <- w36
      n8 = case shown="Default" w28 {
        tunnel: ["A" ("Current Drawing Station") "Current Drawing Station"] -> w29
        tunnel: [TRUE ("Show Flow Data") "Show Flow Data"] -> w26
        frame Default {
        }
        frame "PRAT", "HEWH RLT" {
        }
      }
      n9 = call "HEWH RLT Find TC Channel.vi"("Program Channel Locations In"=T20[] ["021", "022", "023", "024", "025", "026", "017", "028", "029", "030"] ("Array"), "Error In"=w42, "TC Data"=w38, "Station A Channels, MW100"=w37) -> ("Error Out"=w35:errorcluster, "TC Data"=w33:string[][])  [unwired: 6 in]
      n10 = call "HEWH RLT GET Flow Data.vi"("Collect Power Data"=w30, "Error In"=w35, "All Other Data (NO TC's) in"=w36) -> ("Error Out"=w31:errorcluster, "All Other Data (NO TC's) out"=w34:string[][])  [unwired: 7 in]
      n11 = Build Array (concatenate)(w34, w33) -> (w32:string[][])
      n12 = call "HEWH RLT PRAT Data Parse Specific Data.vi"("Data (Label,Data) In"=w32, "Error In"=w31, "Station ID"=w39, "Current Drawing Station"=w29, "Show Flow Data"=w26) -> ("Current (Amps)"=w27:dbl, "Data (Label,Data) Out"=w41:string[][], "Error Out"=w40:errorcluster)  [unwired: 12 in]
    }
  }
  "Data (Label,Data)" <- w10
  "Error Out" <- w8
  "RMS Current (Amps)" <- w3
  "Core HEWH Data Station Output" <- "Core HEWH Data Station A"
